vi "Get Dynamic Panels.vi"(8 "error in (no error)":errorcluster, 11 "PanelArray in":refnum<class "PanelArray.lvclass">) -> (0 "error out":errorcluster, 1 "Heights":i32[](array[numeric]), 2 "Visible Panels":refnum<class "Panel.lvclass">[](array[class]), 3 "PanelArray out":refnum<class "PanelArray.lvclass">)   [LabVIEW 2018, in "OOPanel.lvlib" / "PanelArray.lvclass"]
uses:
  PanelArray.lvclass
  Panel/Panel.lvclass
  PanelArray.lvclass/PanelArray.ctl
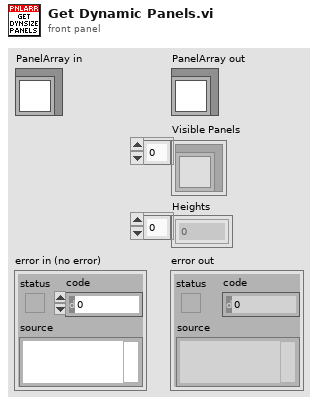
[diagram p1: front panel]
types:
  T1 = typedef "OOPanel.lvlib/PanelArray.lvclass/Ref Data.ctl" = cluster{"State":T2, "Refs":T3, "Events":T4, "Scrolling":T5, "Panels":T6}
  T2 = typedef "OOPanel.lvlib/PanelArray.lvclass/State.ctl" = cluster{"Defer Updates":bool, "Running":bool, "Dynamic Sizing":bool, "Borders":bool}
  T3 = typedef "OOPanel.lvlib/PanelArray.lvclass/Refs.ctl" = cluster{"SubPanels":refnum<vi>[], "Scrollbar":refnum<vi>, "Owning Panel":refnum<vi>}
  T4 = typedef "OOPanel.lvlib/PanelArray.lvclass/Events.ctl" = cluster{"Close":refnum<user-event>}
  T5 = typedef "OOPanel.lvlib/PanelArray.lvclass/Scrolling.ctl" = cluster{"Size":i32, "Max":i32, "Current":i32, "Top Index":i32, "Heights":i32[]}
  T6 = typedef "OOPanel.lvlib/PanelArray.lvclass/Panels.ctl" = cluster{"All":refnum<class "Panel.lvclass">[], "Visible":refnum<class "Panel.lvclass">[], "Blank":refnum<class "ArrayBlank.lvclass">}
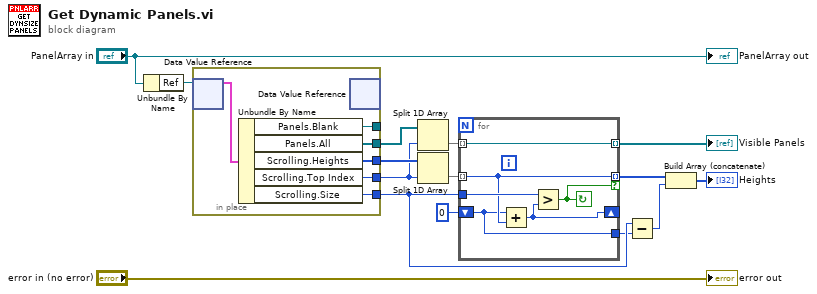
[diagram p0: block diagram]
diagram:
  n1 = Unbundle By Name("PanelArray in") -> ("Ref"=w14:refnum<data-value>)
  n2 = in-place {
    in-place-border: [w20] -> w12
    in-place-border: [w19] -> w10
    in-place-border: [w18] -> w6
    in-place-border: [w17] -> w11
    in-place-border: [w16] -> _
    n3 = in-place-dvr #1(w14) -> (w21:T1)  [unwired: 1 out]
    n4 = Unbundle By Name(w21) -> ("Panels.Blank"=w16:refnum<class "ArrayBlank.lvclass">, "Panels.All"=w17:refnum<class "Panel.lvclass">[], "Scrolling.Heights"=w20:i32[], "Scrolling.Top Index"=w19:i32, "Scrolling.Size"=w18:i32)
    n5 = in-place-dvr #1() -> ()  [unwired: 1 in, 2 out]
  }
  n6 = Split 1D Array(array=w11, index=w10) -> (second subarray=w8:refnum<class "Panel.lvclass">[])  [unwired: 1 out]
  n7 = Split 1D Array(array=w12, index=w10) -> (second subarray=w7:i32[])  [unwired: 1 out]
  n8 = for {
    tunnel: w7 -> [w24] mode=indexing
    tunnel: w6 -> [w27]
    shift-right: [w26] -> _
    shift-left: 0 -> [w22]
    tunnel: w8 -> [w25] mode=indexing
    tunnel: [w25] -> w5 mode=indexing
    tunnel: [w24] -> w4 mode=indexing if=w23
    tunnel: [w22] -> w1
    stop <- w23 continue-if-true
    n9 = Add(x=w22, y=w24) -> (x+y=w26:i32)
    n10 = Greater?(x=w27, y=w26) -> (0:w23:bool)
  }
  "Visible Panels" <- w5
  n11 = Subtract(x=w6, y=w1) -> (x-y=w2:i32)
  n12 = Build Array (concatenate)(w4, w2) -> (→"Heights":i32[])
  "error out" <- "error in (no error)"
  "PanelArray out" <- "PanelArray in"
